vi "arduino_set_init_pressures.vi"(6 "High P":dbl, 8 "error in":errorcluster, 9 "Suction":dbl, 10 "Low P":dbl, 11 "Pressure Box COM in":refnum<visa-resource-name>) -> (0 "error out":errorcluster, 3 "Pressure Box COM out":refnum<visa-resource-name>)   [LabVIEW 2015]
uses:
  pipette cleaning/pressure box/cleaning_soft/controls/arduino_pressure_setting.ctl
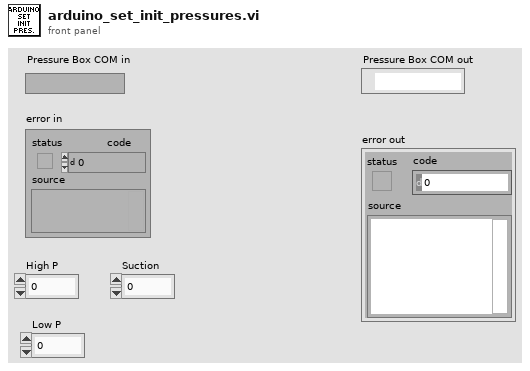
[diagram p1: front panel]
types:
  T1 = typedef "arduino_pressure_setting.ctl" = enum16{"High Positive Pressure", "Low Positive Pressure", "Atmospheric Pressure", "Low Vacuum", "High Vacuum", "Break In", "Puff"}
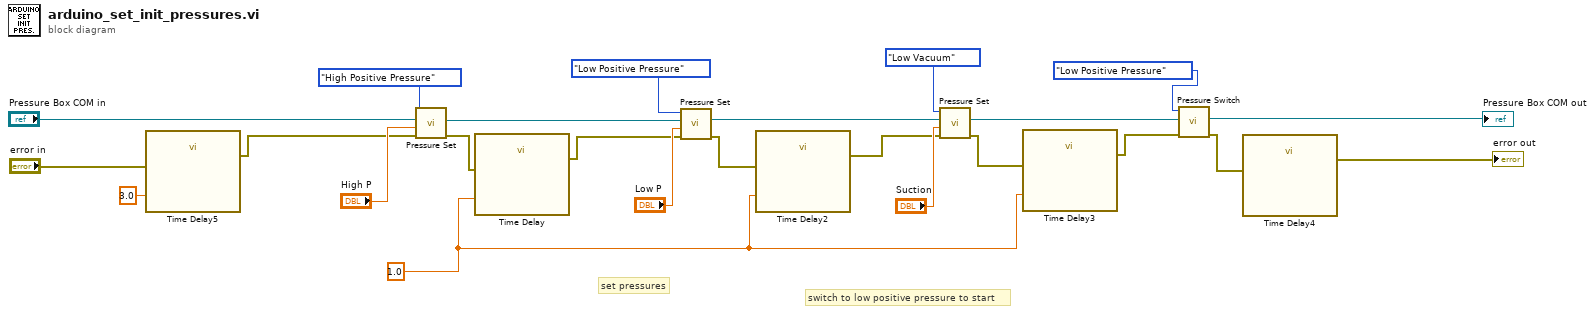
[diagram p0: block diagram]
diagram:
  w10 = 1.0 ("Delay Time (s)")
  # "switch to low positive pressure to start"
  # "set pressures"
  n1 = call "Time Delay5"("error in (no error)"="error in", "Delay Time (s)"=3.0) -> ("error out"=w6:errorcluster)  [unwired: 9 in]
  n2 = call "Pressure Set.vi"("error in"=w6, "Val"="High P", "Pressure Box COM"="Pressure Box COM in", "arduino pressure setting"=arduino_pressure_setting."High Positive Pressure") -> ("error out"=w16:errorcluster, "Pressure Box COM out"=w22:refnum<visa-resource-name>)  [unwired: 6 in]
  n3 = call "Time Delay"("error in (no error)"=w16, "Delay Time (s)"=w10) -> ("error out"=w15:errorcluster)  [unwired: 9 in]
  n4 = call "Pressure Set.vi"("error in"=w15, "Val"="Low P", "Pressure Box COM"=w22, "arduino pressure setting"=arduino_pressure_setting."Low Positive Pressure") -> ("error out"=w14:errorcluster, "Pressure Box COM out"=w23:refnum<visa-resource-name>)  [unwired: 6 in]
  n5 = call "Time Delay2"("error in (no error)"=w14, "Delay Time (s)"=w10) -> ("error out"=w13:errorcluster)  [unwired: 9 in]
  n6 = call "Pressure Set.vi"("error in"=w13, "Val"="Suction", "Pressure Box COM"=w23, "arduino pressure setting"=arduino_pressure_setting."Low Vacuum") -> ("error out"=w12:errorcluster, "Pressure Box COM out"=w18:refnum<visa-resource-name>)  [unwired: 6 in]
  n7 = call "Time Delay3"("error in (no error)"=w12, "Delay Time (s)"=w10) -> ("error out"=w11:errorcluster)  [unwired: 9 in]
  n8 = call "Pressure Switch.vi"("error in"=w11, "Pressure Box COM"=w18, "arduino pressure setting"=arduino_pressure_setting."Low Positive Pressure") -> ("error out"=w9:errorcluster, "Pressure Box COM out"=→"Pressure Box COM out":refnum<visa-resource-name>)  [unwired: 7 in]
  n9 = call "Time Delay4"("error in (no error)"=w9) -> ("error out"=→"error out":errorcluster)  [unwired: 10 in]
